vi "CalculateY1Y2.vi"(8 "error in":errorcluster, 11 "MagSpec_Bella in":refnum<class "MagSpec_Bella.lvclass">) -> (0 "error out":errorcluster, 3 "MagSpec_Bella out":refnum<class "MagSpec_Bella.lvclass">)   [LabVIEW 2020, in "MagSpec_Bella.lvclass"]
uses:
  MagSpec_Bella.lvclass
  Controls/CameraSettings_File.ctl
  MagSpec_Bella.lvclass/MagSpec_Bella.ctl
  shared/OnOffTypeDef.ctl
  Controls/Calibration_Pixel_based.ctl
panel:
  out "Waveform Graph 4":dbl[][](graph)
  out "Camera Settings 2":T1
  out "y2":dbl[](graph)
  out "y1":dbl[](graph)
  out "Waveform Graph 2":dbl[][](graph)
  out "Array":dbl[][](array[numeric])
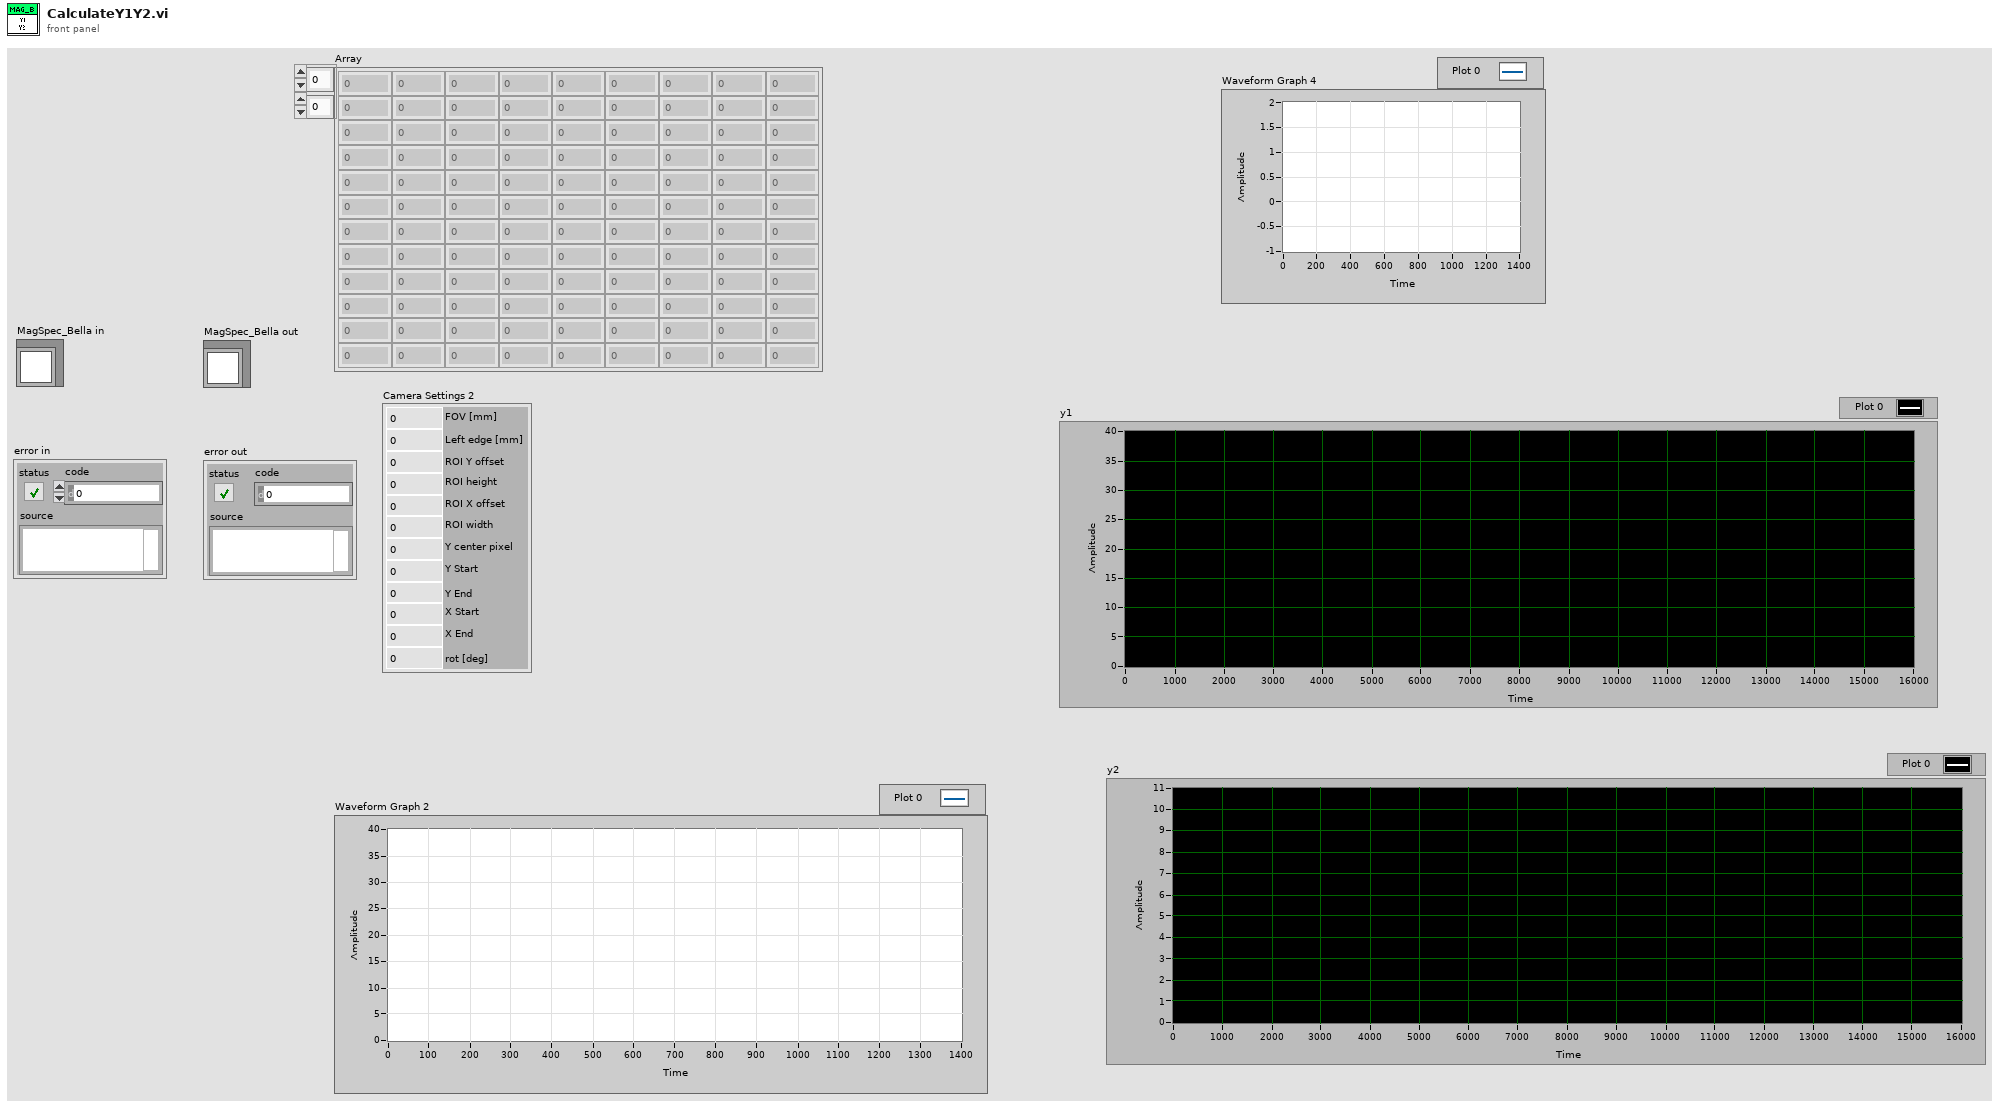
[diagram p1: front panel]
types:
  T1 = typedef "CameraSettings_File.ctl" = cluster{"FOV [mm]":dbl, "Left edge [mm]":dbl, "ROI Y offset":dbl, "ROI height":dbl, "ROI X offset":dbl, "ROI width":dbl, "Y center pixel":dbl, "Y Start":dbl, "Y End":dbl, "X Start":dbl, "X End":dbl, "rot [deg]":dbl}
  T2 = typedef "OneTimeCalculation.ctl" = cluster{"first Pixel pos [m]":dbl, "Pixel Size [mm]":dbl, "forward":T3}
  T3 = typedef "OnOffTypeDef.ctl" = enum16{"off", "on"}
  T4 = typedef "CalibrationCluster.ctl" = cluster{"bending angle Front":dbl[], "bending angle Side":dbl[], "screen [m] Front":dbl[], "screen [m] Side":dbl[], "momentum [MeV/c]":dbl[], "total path [m]":dbl[], "x[mm](rms)":dbl[], "x[mm](rms,b)":dbl[], "y[mm](rms)":dbl[], "y[mm](rms,b)":dbl[]}
  T5 = typedef "Calibration_Pixel_based.ctl" = cluster{"y1(pixel)":dbl[], "y2(pixel)":dbl[], "dp/B [MeV/C/B] (pixel)":dbl[], "energyDependence Input(pixel)":dbl[], "bending angle [deg](pixel)":dbl[], "total path(pixel)":dbl[], "pixel angle (y)(pixel)":dbl[], "energy dependence (pixel)":dbl[], "charge compensation (pixel)":dbl[], "Momentum [MeV/C](pixel)":dbl[], "angular compensation(pixel)":dbl[]}
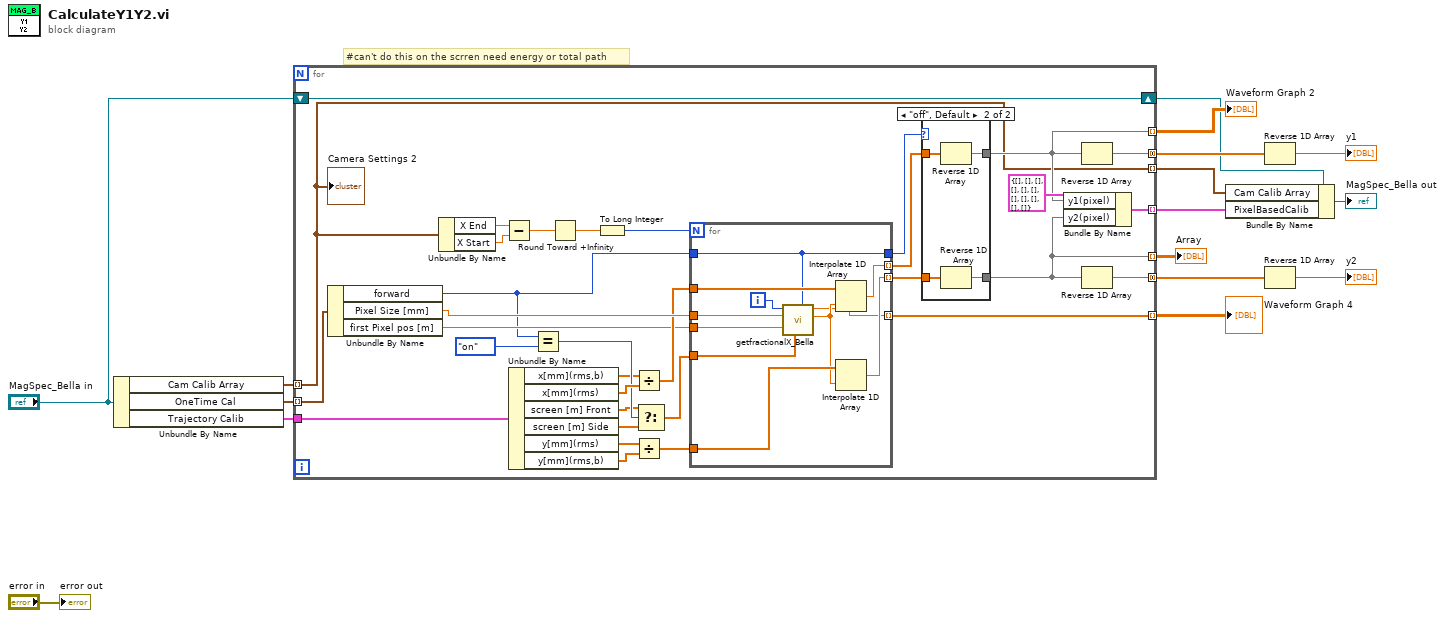
[diagram p0: block diagram]
diagram:
  # "#can't do this on the scrren need energy or total path"
  n1 = Unbundle By Name("MagSpec_Bella in") -> ("Cam Calib Array"=w11:T1[], "OneTime Cal"=w13:T2[], "Trajectory Calib"=w14:T4)
  n2 = for {
    tunnel: w13 -> [w45] mode=indexing
    tunnel: w14 -> [w43]
    tunnel: [w37] -> w15 mode=indexing
    tunnel: w11 -> [w23] mode=indexing
    tunnel: [w29] -> w5 mode=indexing
    tunnel: [w31] -> w10 mode=indexing
    tunnel: [w30] -> w7 mode=concatenating
    tunnel: [w28] -> w9 mode=concatenating
    shift-right: [w26] -> w3
    shift-left: "MagSpec_Bella in" -> [w26]
    tunnel: [w23] -> w2 mode=indexing
    tunnel: [w21] -> w1 mode=indexing
    n3 = Unbundle By Name(w45) -> ("forward"=w17:T3, "Pixel Size [mm]"=w44:dbl, "first Pixel pos [m]"=w22:dbl)
    n4 = Unbundle By Name(w23) -> ("X End"=w39:dbl, "X Start"=w38:dbl)
    n5 = Subtract(x=w39, y=w38) -> (x-y=w20:dbl)
    n6 = Unbundle By Name(w43) -> ("x[mm](rms,b)"=w36:dbl[], "x[mm](rms)"=w46:dbl[], "screen [m] Front"=w35:dbl[], "screen [m] Side"=w34:dbl[], "y[mm](rms)"=w49:dbl[], "y[mm](rms,b)"=w48:dbl[])
    n7 = Equal?(x=w17, y=OnOffTypeDef."on") -> (x = y?=w41:bool)
    n8 = Round Toward +Infinity(x=w20) -> (ceil(x): smallest int >= x=w19:dbl)
    n9 = To Long Integer(number=w19) -> (32bit integer=w18:i32)
    n10 = Divide(x=w36, y=w46) -> (x/y=w33:dbl[])
    n11 = Divide(x=w49, y=w48) -> (x/y=w47:dbl[])
    n12 = Select(t=w35, s=w41, f=w34) -> (s? t:f=w32:dbl[])
    n13 = for {
      N: w18 -> [_]
      tunnel: w32 -> [w60]
      tunnel: w44 -> [w62]
      tunnel: w22 -> [w61]
      tunnel: w33 -> [w66]
      tunnel: w47 -> [w65]
      tunnel: [w64] -> w24 mode=indexing
      tunnel: [w63] -> w25 mode=indexing
      tunnel: w17 -> [w57]
      tunnel: [w57] -> w27
      tunnel: [w56] -> w21 mode=indexing
      i -> [w58]
      n14 = call "getfractionalX_Bella.vi"("CameraFlipped"=w57, "screen [m]"=w60, "position [m]"=w61, "pixelsize"=w62, "position index"=w58) -> ("index"=w59:dbl, "position m"=w56:dbl)  [unwired: 5 in]
      n15 = Interpolate 1D Array(1:w59, 2:w66) -> (0:w64:dbl)
      n16 = Interpolate 1D Array(1:w59, 2:w65) -> (0:w63:dbl)
    }
    n17 = case shown="\"off\", Default" w27 {
      tunnel: [w50 w55] -> w31
      tunnel: w24 -> [w50 w54]
      tunnel: [w51 w53] -> w29
      tunnel: w25 -> [w51 w52]
      frame "on" {
      }
      frame "off", Default {
        n18 = Reverse 1D Array(array=w54) -> (reversed array=w55:dbl[])
        n19 = Reverse 1D Array(array=w52) -> (reversed array=w53:dbl[])
      }
    }
    n20 = Bundle By Name(cluster=T5 {"y1(pixel)"=[], "y2(pixel)"=[], "dp/B [MeV/C/B] (pixel)"=[], "energyDependence Input(pixel)"=[], "bending angle [deg](pixel)"=[], "total path(pixel)"=[], "pixel angle (y)(pixel)"=[], "energy dependence (pixel)"=[], "charge compensation (pixel)"=[], "Momentum [MeV/C](pixel)"=[], "angular compensation(pixel)"=[]} ("Cluster"), "y1(pixel)"=w31, "y2(pixel)"=w29) -> (w37:T5)
    n21 = Reverse 1D Array(array=w31) -> (reversed array=w30:dbl[])
    n22 = Reverse 1D Array(array=w29) -> (reversed array=w28:dbl[])
    "Camera Settings 2" <- w23
  }
  "Array" <- w5
  "Waveform Graph 2" <- w10
  "Waveform Graph 4" <- w1
  n23 = Bundle By Name(cluster=w3, "Cam Calib Array"=w2, "PixelBasedCalib"=w15) -> (→"MagSpec_Bella out":refnum<class "MagSpec_Bella.lvclass">)
  n24 = Reverse 1D Array(array=w7) -> (reversed array=→"y1":dbl[])
  n25 = Reverse 1D Array(array=w9) -> (reversed array=→"y2":dbl[])
  "error out" <- "error in"
